vi "Order Patterns.vi"(8 "error in (no error)":errorcluster, 10 "Lithography Data":T1(array[cluster]), 11 "ListBox Reference in":refnum<vi>) -> (0 "error out":errorcluster, 3 "Ordered Lithography Data":T1(array[cluster]))   [LabVIEW 2016]
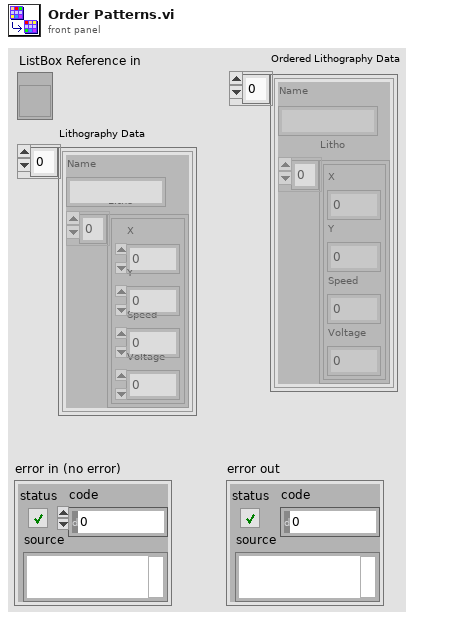
[diagram p1: front panel]
types:
  T1 = cluster{"Name":string, "Litho":cluster{"X":dbl, "Y":dbl, "Speed":dbl, "Voltage":dbl}[]}[]
  T2 = cluster{"Name":string, "Litho":cluster{"X":dbl, "Y":dbl, "Speed":dbl, "Voltage":dbl}[]}
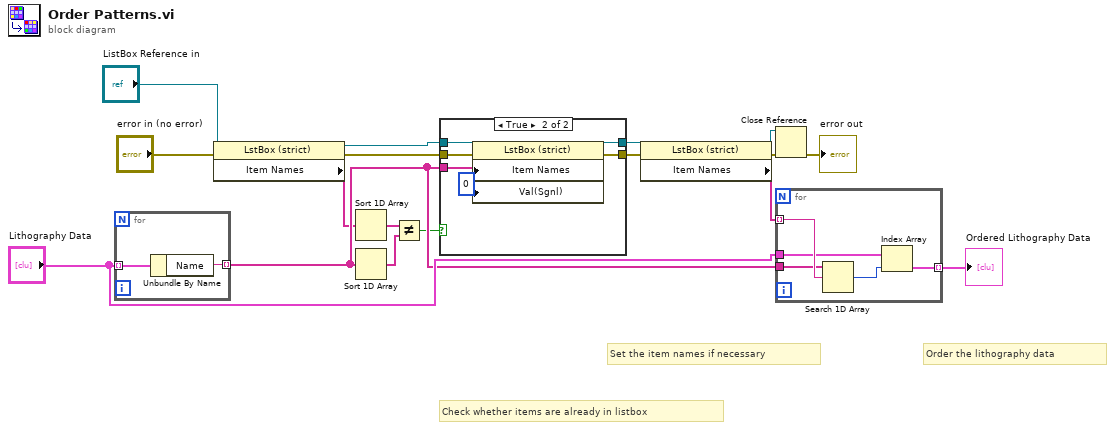
[diagram p0: block diagram]
diagram:
  # "Check whether items are already in listbox"
  # "Set the item names if necessary"
  # "Order the lithography data"
  n1 = for {
    tunnel: "Lithography Data" -> [w19] mode=indexing
    tunnel: [w18] -> w15 mode=indexing
    n2 = Unbundle By Name(w19) -> ("Name"=w18:string)
  }
  n3 = property class="LstBox (strict)"(reference="ListBox Reference in", error in="error in (no error)") -> (reference out=w5:refnum<vi>, error out=w6:errorcluster, "Item Names"=w2:string[])
  n4 = Sort 1D Array(array=w2) -> (sorted array=w7:string[])
  n5 = Sort 1D Array(array=w15) -> (sorted array=w8:string[])
  n6 = Not Equal?(x=w7, y=w8) -> (x != y?=w3:bool)
  n7 = case shown="True" w3 {
    tunnel: w15 -> [_ w27]
    tunnel: w5 -> [w21 w26]
    tunnel: w6 -> [w20 w25]
    tunnel: [w20 w24] -> w13
    tunnel: [w21 w23] -> w12
    frame False {
    }
    frame True {
      n8 = property class="LstBox (strict)"(reference=w26, error in=w25, "Item Names"=w27, "Val(Sgnl)"=0 ("Value (Signaling)")) -> (reference out=w23:refnum<vi>, error out=w24:errorcluster)
    }
  }
  n9 = property class="LstBox (strict)"(reference=w12, error in=w13) -> (reference out=w9:refnum<vi>, error out=w10:errorcluster, "Item Names"=w14:string[])
  n10 = Close Reference(reference=w9, error in (no error)=w10) -> (error out=→"error out":errorcluster)
  n11 = for {
    tunnel: w14 -> [w32] mode=indexing
    tunnel: w15 -> [w30]
    tunnel: [w29] -> w17 mode=indexing
    tunnel: "Lithography Data" -> [w28]
    n12 = Search 1D Array(1D array=w30, element=w32) -> (index of element=w31:i32)  [unwired: 1 in]
    n13 = Index Array(array=w28, index=w31) -> (element=w29:T2)
  }
  "Ordered Lithography Data" <- w17
